vi "Burst Apply (G3).vi"(6 "Duplicate?":bool, 8 "error in (no error)":errorcluster, 9 "Waveform in":dbl[](array[numeric]), 10 "Sampling Rate (Hz)":dbl, 11 "Burst":T1) -> (0 "error out":errorcluster, 1 "Gated waveform":dbl[](array[numeric]))   [LabVIEW 2020]
uses:
  Controls/Burst XCtl/Burst Data.ctl
  Controls/Burst XCtl/Burst Control.xctl
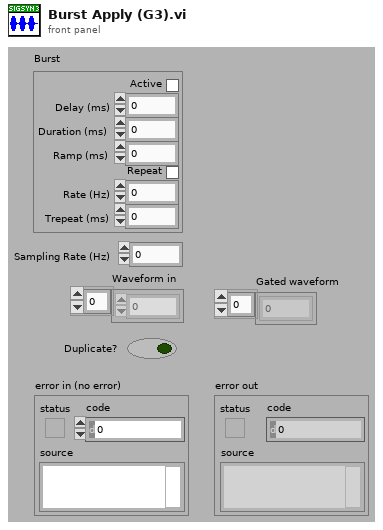
[diagram p1: front panel]
types:
  T1 = typedef "Burst Control.xctl/Burst Data.ctl" = cluster{"Active":bool, "Delay (ms)":dbl, "Duration (ms)":dbl, "Ramp (ms)":dbl, "Rate (Hz)":dbl, "Trepeat (ms)":dbl, "Repeat":bool}
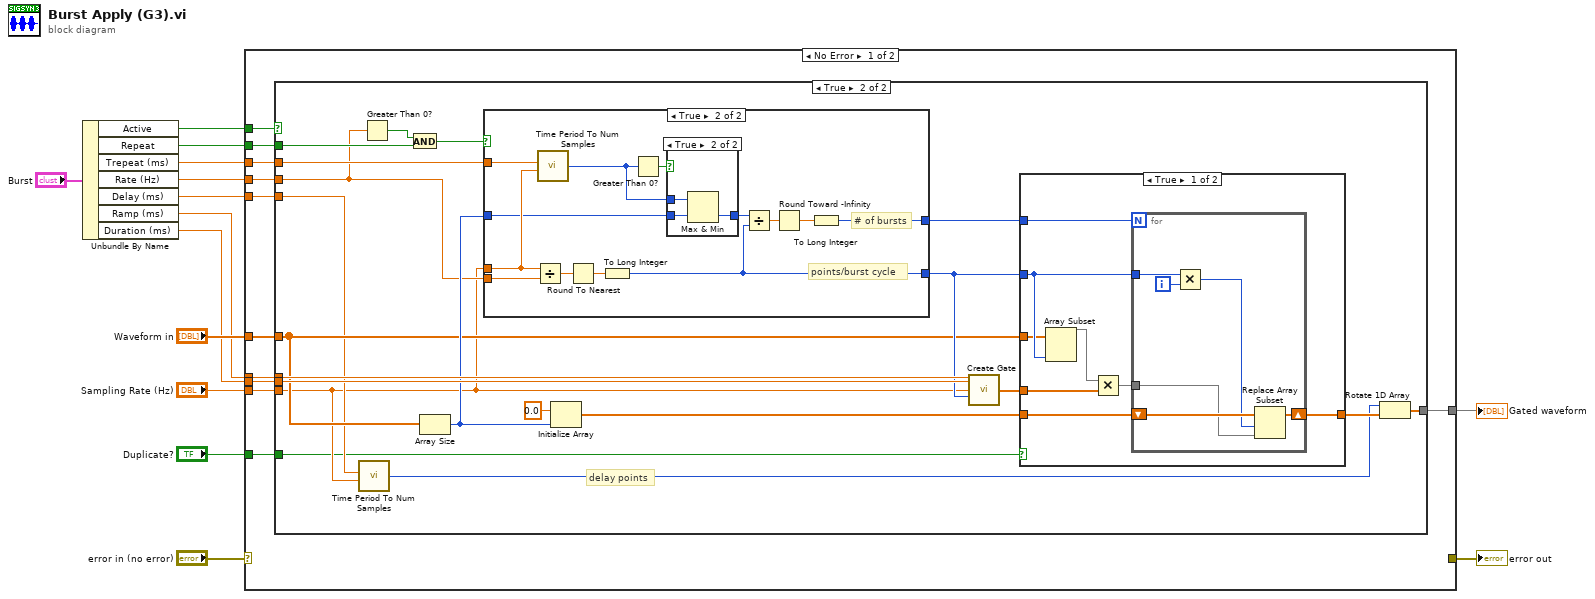
[diagram p0: block diagram]
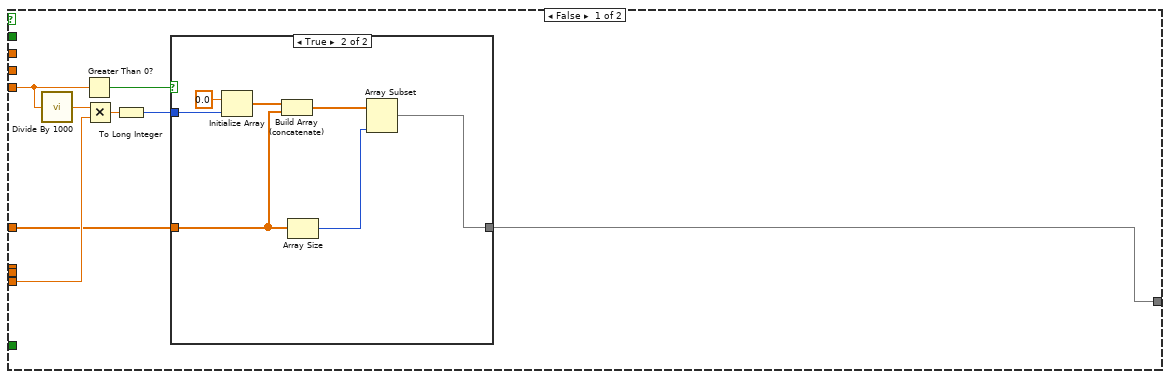
[diagram p2: hidden frame]
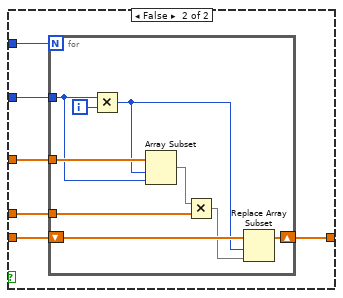
[diagram p4: hidden frame]
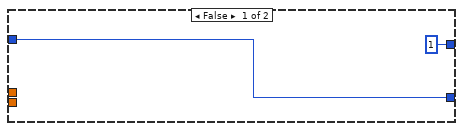
[diagram p5: hidden frame]
diagram:
  n1 = Unbundle By Name("Burst") -> ("Active"=w12:bool, "Repeat"=w9:bool, "Trepeat (ms)"=w8:dbl, "Rate (Hz)"=w4:dbl, "Delay (ms)"=w2:dbl, "Ramp (ms)"=w6:dbl, "Duration (ms)"=w5:dbl)
  n2 = case shown="No Error" "error in (no error)" {
    selector: "error in (no error)" -> [_ w110]
    tunnel: w12 -> [w16 _]
    tunnel: "Waveform in" -> [w22 _]
    tunnel: [_ w110] -> w10
    tunnel: w6 -> [w24 _]
    tunnel: w5 -> [w23 _]
    tunnel: w9 -> [w25 _]
    tunnel: "Sampling Rate (Hz)" -> [w18 _]
    tunnel: w8 -> [w17 _]
    tunnel: [w21 _] -> w7
    tunnel: w4 -> [w20 _]
    tunnel: w2 -> [w19 _]
    tunnel: "Duplicate?" -> [w15 _]
    frame No Error {
      n3 = case shown="True" w16 {
        tunnel: w25 -> [_ w50]
        tunnel: w24 -> [_ w61]
        tunnel: w23 -> [_ w60]
        tunnel: w17 -> [_ w51]
        tunnel: w22 -> [w29 w53]
        tunnel: [w26 w47] -> w21
        tunnel: w20 -> [_ w49]
        tunnel: w19 -> [w33 w45]
        tunnel: w18 -> [w31 w44]
        tunnel: w15 -> [_ w42]
        frame False {
          n4 = call "Divide By 1000.vi"("X"=w33) -> ("X/1000"=w32:dbl)
          n5 = Greater Than 0?(x=w33) -> (x > 0?=w28:bool)
          n6 = Multiply(x=w32, y=w31) -> (x*y=w30:dbl)
          n7 = To Long Integer(number=w30) -> (32bit integer=w27:i32)
          n8 = case shown="True" w28 {
            tunnel: w29 -> [w34 w37]
            tunnel: w27 -> [_ w41]
            tunnel: [w34 w35] -> w26
            frame False {
            }
            frame True {
              n9 = Initialize Array(0.0 ("element"), w41) -> (w39:dbl[])
              n10 = Build Array (concatenate)(w39, w37) -> (w38:dbl[])
              n11 = Array Size(array=w37) -> (size(s)=w36:i32)
              n12 = Array Subset(array=w38, length=w36) -> (w35:dbl[])  [unwired: 1 in]
            }
          }
        }
        frame True {
          # "delay points"
          n13 = call "Time Period To Num Samples.vi"("Duration (ms)"=w45, "Sampling rate (Hz)"=w44) -> ("Samples"=w43:i32)  [unwired: 5 in]
          n14 = Greater Than 0?(x=w49) -> (x > 0?=w52:bool)
          n15 = And(x=w52, y=w50) -> (x .and. y?=w48:bool)
          n16 = Array Size(array=w53) -> (size(s)=w59:i32)
          n17 = case shown="True" w48 {
            tunnel: w59 -> [w92 w93]
            tunnel: w44 -> [_ w96]
            tunnel: [w92 w102] -> w54
            tunnel: w51 -> [_ w95]
            tunnel: [1 w99] -> w57
            tunnel: w49 -> [_ w98]
            frame False {
            }
            frame True {
              # "# of bursts"
              # "points/burst cycle"
              n18 = Divide(x=w96, y=w98) -> (x/y=w105:dbl)
              n19 = call "Time Period To Num Samples.vi"("Duration (ms)"=w95, "Sampling rate (Hz)"=w96) -> ("Samples"=w94:i32)  [unwired: 5 in]
              n20 = Round To Nearest(number=w105) -> (nearest integer value=w104:dbl)
              n21 = To Long Integer(number=w104) -> (32bit integer=w102:i32)
              n22 = Greater Than 0?(x=w94) -> (x > 0?=w97:bool)
              n23 = case shown="True" w97 {
                tunnel: w94 -> [_ w109]
                tunnel: [w106 w108] -> w103
                tunnel: w93 -> [w106 w107]
                frame False {
                }
                frame True {
                  n24 = Max & Min(x=w109, y=w107) -> (min(x,y)=w108:i32)  [unwired: 1 out]
                }
              }
              n25 = Divide(x=w103, y=w102) -> (x/y=w101:dbl)
              n26 = Round Toward -Infinity(1:w101) -> (0:w100:dbl)
              n27 = To Long Integer(number=w100) -> (32bit integer=w99:i32)
            }
          }
          n28 = Initialize Array(0.0 ("element"), w59) -> (w55:dbl[])
          n29 = call "Create Gate.vi"("Ramp (ms)"=w61, "Duration (ms)"=w60, "Sampling Rate (Hz)"=w44, "Npts"=w54) -> ("Gate"=w56:dbl[])  [unwired: 10 in, 1 out]
          n30 = case shown="True" w42 {
            tunnel: w57 -> [w69 w81]
            tunnel: w56 -> [w68 w77]
            tunnel: w55 -> [w67 w80]
            tunnel: w54 -> [w66 w79]
            tunnel: w53 -> [w65 w76]
            tunnel: [w62 w78] -> w46
            frame True {
              n31 = Array Subset(array=w65, length=w66) -> (w63:dbl[])  [unwired: 1 in]
              n32 = Multiply(x=w63, y=w68) -> (x*y=w64:dbl[])
              n33 = for {
                N: w69 -> [_]
                tunnel: w64 -> [w73]
                shift-right: [w74] -> w62
                shift-left: w67 -> [w75]
                tunnel: w66 -> [w71]
                i -> [w72]
                n34 = Multiply(x=w71, y=w72) -> (x*y=w70:i32)
                n35 = Replace Array Subset(array=w75, new element=w73, index=w70) -> (w74:dbl[])
              }
            }
            frame False {
              n36 = for {
                N: w81 -> [_]
                shift-right: [w89] -> w78
                shift-left: w80 -> [w90]
                tunnel: w79 -> [w83]
                tunnel: w77 -> [w87]
                tunnel: w76 -> [w85]
                i -> [w88]
                n37 = Multiply(x=w83, y=w88) -> (x*y=w84:i32)
                n38 = Array Subset(array=w85, index=w84, length=w83) -> (w82:dbl[])
                n39 = Multiply(x=w82, y=w87) -> (x*y=w86:dbl[])
                n40 = Replace Array Subset(array=w90, new element=w86, index=w84) -> (w89:dbl[])
              }
            }
          }
          n41 = Rotate 1D Array(1:w46, 2:w43) -> (0:w47:dbl[])
        }
      }
    }
    frame Error {
    }
  }
  "error out" <- w10
  "Gated waveform" <- w7
